vi "Log Data.vi"(8 "error in (no error)":errorcluster, 10 "Data Queue":refnum<queue>, 11 "Logging Configuration":T1) -> (0 "error out":errorcluster)   [LabVIEW 2022 SP3, in "Logging.lvlib"]
doc: "This VI uses the TDMS Write function to write data to a TDMS file."
uses:
  Logging.lvlib
  Logging Configuration.ctl
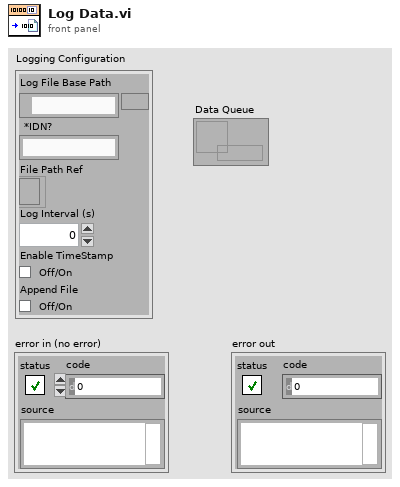
[diagram p1: front panel]
types:
  T1 = typedef "Logging.lvlib/Logging Configuration.ctl" = cluster{"Log File Base Path":path, "*IDN?":string, "File Path Ref":refnum<file>, "Log Interval (s)":dbl, "Enable TimeStamp":bool, "Append File":bool}
  T2 = enum16{"open", "replace", "create", "open or create", "replace or create", "replace or create with confirmation"}
  T3 = cluster{"Numeric":dbl, "Numeric":dbl, "Numeric":dbl, timestamp}
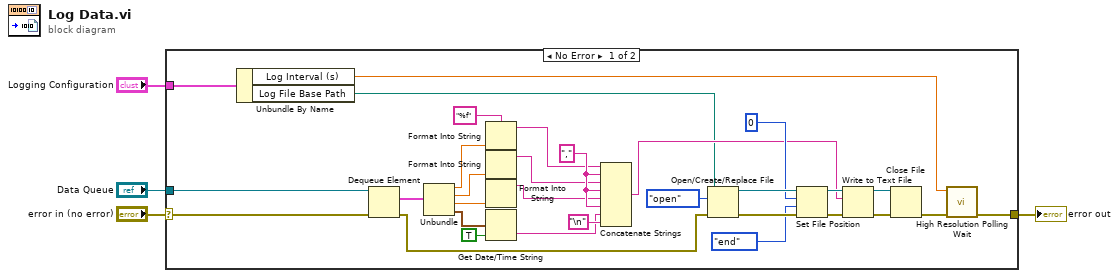
[diagram p0: block diagram]
diagram:
  n1 = case shown="No Error" "error in (no error)" {
    selector: "error in (no error)" -> [w34 w36]
    tunnel: "Logging Configuration" -> [w35 _]
    tunnel: [w6 w36] -> w3
    tunnel: "Data Queue" -> [w33 _]
    frame No Error {
      w18 = ","
      w14 = "%f"
      n2 = Unbundle By Name(w35) -> ("Log Interval (s)"=w5:dbl, "Log File Base Path"=w12:path)
      n3 = Dequeue Element(queue=w33, error in (no error)=w34) -> (element=w32:T3, error out=w11:errorcluster)  [unwired: 1 in, 2 out]
      n4 = Unbundle(w32) -> ("Numeric"=w19:dbl, "Numeric"=w20:dbl, "Numeric"=w21:dbl, w10:timestamp)
      n5 = Format Into String(format string=w14, w19) -> (resulting string=w17:string)  [unwired: 2 in, 1 out]
      n6 = Format Into String(format string=w14, w20) -> (resulting string=w16:string)  [unwired: 2 in, 1 out]
      n7 = Format Into String(format string=w14, w21) -> (resulting string=w15:string)  [unwired: 2 in, 1 out]
      n8 = Get Date/Time String(seconds (now)=w10, want seconds? (F)=TRUE) -> (time string=w8:string)  [unwired: 1 in, 1 out]
      n9 = Concatenate Strings(w17, w18, w16, w18, w15, w18, w8, "\n") -> (w22:string)
      n10 = Open/Create/Replace File(file path (use dialog)=w12, error in=w11, operation (0:open)=T2."open") -> (refnum out=w28:refnum<file>, error out=w26:errorcluster)  [unwired: 3 in, 1 out]
      n11 = Set File Position(offset (in bytes) (0)=i64 0, refnum=w28, from (0:start)=enum16{"start", "end", "current"}."end", error in=w26) -> (refnum out=w27:refnum<file>, error out=w25:errorcluster)
      n12 = Write to Text File(file (use dialog)=w27, text=w22, error in=w25) -> (refnum out=w30:refnum<file>, error out=w31:errorcluster)  [unwired: 1 in, 1 out]
      n13 = Close File(refnum=w30, error in=w31) -> (error out=w7:errorcluster)  [unwired: 1 out]
      n14 = call <vilib>:"High Resolution Polling Wait.vi"("error in (no error)"=w7, "seconds to wait"=w5) -> ("error out"=w6:errorcluster)  [unwired: 9 in]
    }
    frame Error {
    }
  }
  "error out" <- w3
